vi "Set Custom Device Driver VIs.vi"(8 "error in (no error)":errorcluster, 10 "Driver VIs":T1[](array[typedef]) {"Type" items=["Absolute", "ToBase", "ToCommonDocDir", "ToApplicationDataDir"]}, 11 "BaseNodeType":refnum<k24>) -> (0 "error out":errorcluster, 3 "BaseNodeType out":refnum<k24>)   [LabVIEW 2017, in "VeriStand SLSC Scripting.lvlib"]
uses:
  VeriStand SLSC Scripting.lvlib
  Controls/Driver VI Information.ctl
  <vilib>/NI Veristand/Custom Device API/Custom Device Supported Target.ctl
  NationalInstruments.VeriStand.SystemStorage
  <vilib>/NI Veristand/Custom Device API/Custom Device API.lvlib
panel:
  in  "SupportedTarget":i32(ring) items=["All", "Pharlap", "VxWorks", "Windows", "Linux_32_ARM", "Linux_x64", "PharlapWindows", "PharlapVxWorks", "VxWorksWindows"]
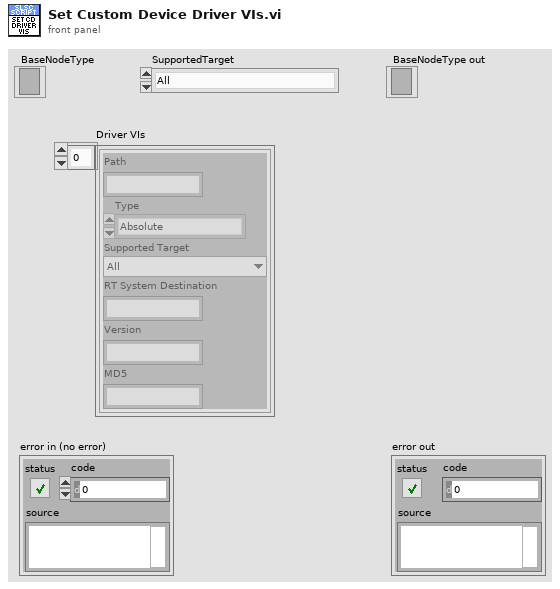
[diagram p1: front panel]
types:
  T1 = typedef "VeriStand SLSC Scripting.lvlib/Driver VI Information.ctl" = cluster{"Path":string, "Type":i32, "Supported Target":T2, "RT System Destination":string, "Version":string, "MD5":string}
  T2 = typedef "Custom Device API.lvlib/Custom Device Supported Target.ctl" = enum16{"All", "PharLap", "VxWorks", "Windows", "Linux_32_ARM", "Linux_x64", "PharLap & Windows", "PharLap & VxWorks", "VxWorks & Windows"}
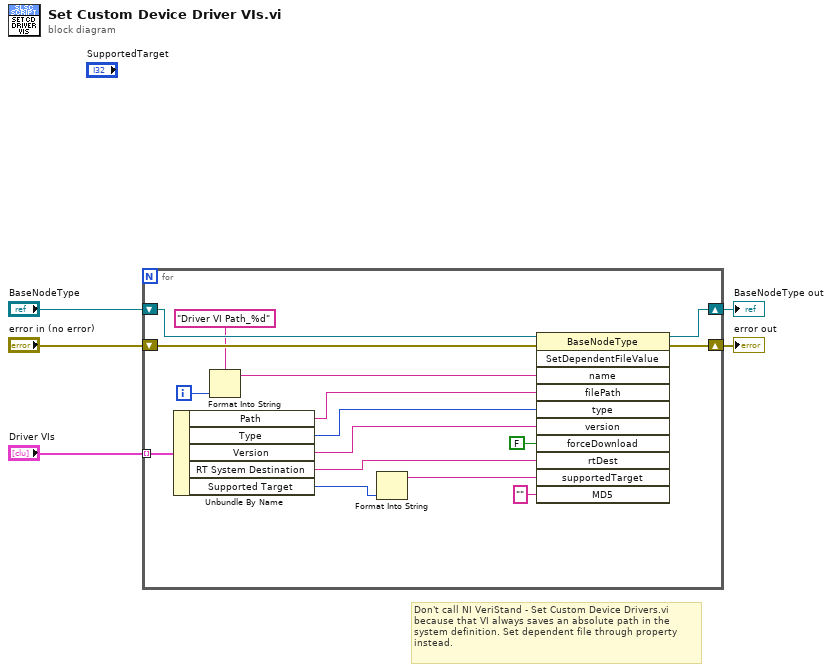
[diagram p0: block diagram]
diagram:
  # "Don't call NI VeriStand - Set Custom Device Drivers.vi\nbecause that VI always saves an absolute path in the\nsystem definition. Set dependent file through property\ninstead."
  n1 = for {
    shift-right: [w18] -> w2
    shift-left: "error in (no error)" -> [w21]
    shift-right: [w19] -> w1
    shift-left: "BaseNodeType" -> [w20]
    tunnel: "Driver VIs" -> [w17] mode=indexing
    i -> [w16]
    n2 = Unbundle By Name(w17) -> ("Path"=w14:string, "Type"=w13:i32, "Version"=w12:string, "RT System Destination"=w10:string, "Supported Target"=w7:T2)
    n3 = Format Into String(format string="Driver VI Path_%d", w16) -> (resulting string=w15:string)  [unwired: 2 in, 1 out]
    n4 = Format Into String(w7) -> (resulting string=w6:string)  [unwired: 3 in, 1 out]
    n5 = invoke class="BaseNodeType" method="SetDependentFileValue"(reference=w20, error in=w21, "name"=w15, "filePath"=w14, "type"=w13, "version"=w12, "forceDownload"=FALSE, "rtDest"=w10, "supportedTarget"=w6, "MD5"="") -> (reference out=w19:refnum<k24>, error out=w18:errorcluster)  [unwired: 1 in, 9 out]
  }
  "error out" <- w2
  "BaseNodeType out" <- w1
